vi "subVI Write to Exfo.vi"(2 "error in":errorcluster, 3 "Command Parameter":u16, 4 "Command Number":u8, 5 "VISA Resource Name":refnum<visa-resource-name>) -> (0 "error out":errorcluster, 1 "dup VISA resource name":refnum<visa-resource-name>)   [LabVIEW 2012]
panel:
  # "Output from subVI"
  # "Inputs to SubVI"
  # "1  =  Connect\n2  =  Lock Front Panel\n3  =  Unlock Front Panel\n4  =  Get Software Version\n5  =  Get Lamp Hours\n6  =  Get Unit Status\n7  =  Clear Alarm\n8  =  Run Timed Exposure\n9  =  Open Shutter\n10 = Close Shutter\n11 = Get Intensity Level\n12  = Set Intensity level\n13 = Get Exposure Level\n14 = Set Exposure Time\n15 = Turn Lamp ON\n16 = Turn Lamp OFF"
  # "0, 1, 2, 3 or 4\n \nseconds * 10"
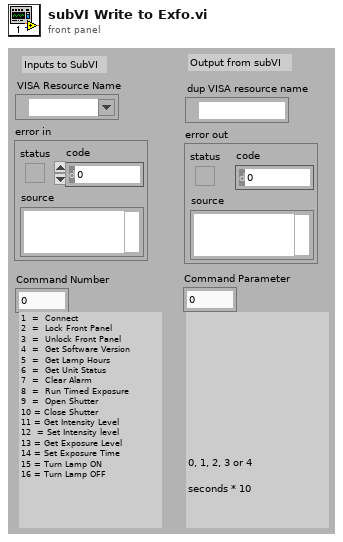
[diagram p1: front panel]
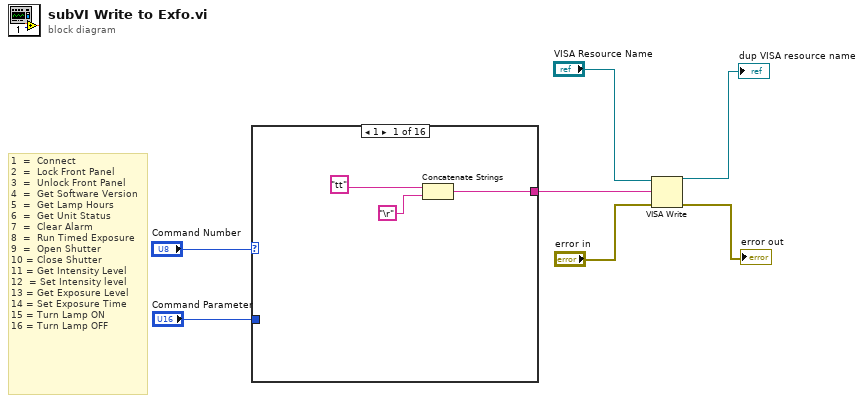
[diagram p0: block diagram]
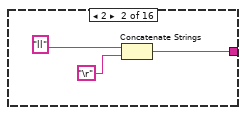
[diagram p2: hidden frame]
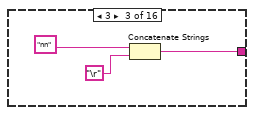
[diagram p3: hidden frame]
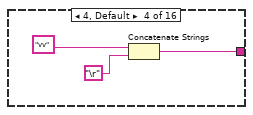
[diagram p4: hidden frame]
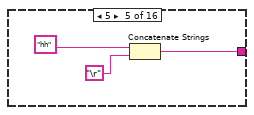
[diagram p5: hidden frame]
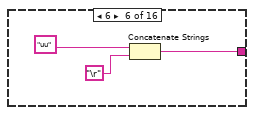
[diagram p6: hidden frame]
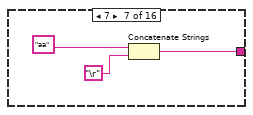
[diagram p7: hidden frame]
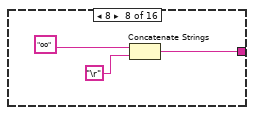
[diagram p8: hidden frame]
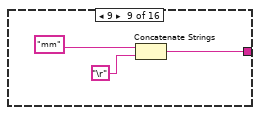
[diagram p9: hidden frame]
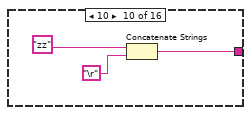
[diagram p10: hidden frame]
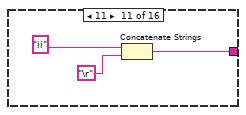
[diagram p11: hidden frame]
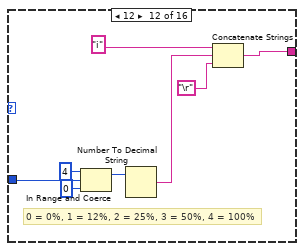
[diagram p12: hidden frame]
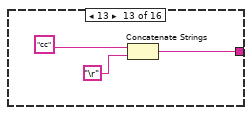
[diagram p13: hidden frame]
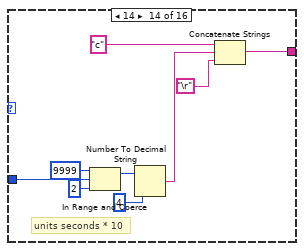
[diagram p14: hidden frame]
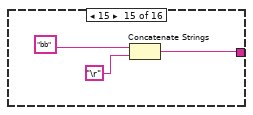
[diagram p15: hidden frame]
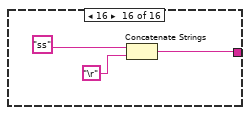
[diagram p16: hidden frame]
diagram:
  # "1  =  Connect\n2  =  Lock Front Panel\n3  =  Unlock Front Panel\n4  =  Get Software Version\n5  =  Get Lamp Hours\n6  =  Get Unit Status\n7  =  Clear Alarm\n8  =  Run Timed Exposure\n9  =  Open Shutter\n10 = Close Shutter\n11 = Get Intensity Level\n12  = Set Intensity level\n13 = Get Exposure Level\n14 = Set Exposure Time\n15 = Turn Lamp ON\n16 = Turn Lamp OFF"
  n1 = case shown="1" "Command Number" {
    tunnel: [w8 w11 w14 w17 w20 w23 w26 w29 w32 w35 w38 w47 w49 w59 w61 w64] -> w4
    tunnel: "Command Parameter" -> [_ _ _ _ _ _ _ _ _ _ _ w46 _ w55 _ _]
    frame 1 {
      n2 = Concatenate Strings("tt" ("string"), "\r") -> (w8:string)
    }
    frame 2 {
      n3 = Concatenate Strings("ll" ("string"), "\r") -> (w11:string)
    }
    frame 3 {
      n4 = Concatenate Strings("nn" ("string"), "\r") -> (w14:string)
    }
    frame 4, Default {
      n5 = Concatenate Strings("vv" ("string"), "\r") -> (w17:string)
    }
    frame 5 {
      n6 = Concatenate Strings("hh" ("string"), "\r") -> (w20:string)
    }
    frame 6 {
      n7 = Concatenate Strings("uu" ("string"), "\r") -> (w23:string)
    }
    frame 7 {
      n8 = Concatenate Strings("aa" ("string"), "\r") -> (w26:string)
    }
    frame 8 {
      n9 = Concatenate Strings("oo" ("string"), "\r") -> (w29:string)
    }
    frame 9 {
      n10 = Concatenate Strings("mm" ("string"), "\r") -> (w32:string)
    }
    frame 10 {
      n11 = Concatenate Strings("zz" ("string"), "\r") -> (w35:string)
    }
    frame 11 {
      n12 = Concatenate Strings("ii" ("string"), "\r") -> (w38:string)
    }
    frame 12 {
      # "0 = 0%, 1 = 12%, 2 = 25%, 3 = 50%, 4 = 100%"
      n13 = In Range and Coerce(upper limit=u8 4, x=w46, lower limit=u8 0) -> (coerced(x)=w43:u16)  [unwired: 1 out]
      n14 = Number To Decimal String(number=w43) -> (decimal integer string=w42:string)  [unwired: 1 out]
      n15 = Concatenate Strings("i" ("string"), w42, "\r") -> (w47:string)
    }
    frame 13 {
      n16 = Concatenate Strings("cc" ("string"), "\r") -> (w49:string)
    }
    frame 14 {
      # "units seconds * 10"
      n17 = In Range and Coerce(upper limit=u16 9999, x=w55, lower limit=u16 2) -> (coerced(x)=w58:u16)  [unwired: 1 out]
      n18 = Number To Decimal String(number=w58, width (-)=i16 4) -> (decimal integer string=w57:string)
      n19 = Concatenate Strings("c" ("string"), w57, "\r") -> (w59:string)
    }
    frame 15 {
      n20 = Concatenate Strings("bb" ("string"), "\r") -> (w61:string)
    }
    frame 16 {
      n21 = Concatenate Strings("ss" ("string"), "\r") -> (w64:string)
    }
  }
  n22 = VISA Write(VISA resource name="VISA Resource Name", write buffer=w4, error in (no error)="error in") -> (VISA resource name out=→"dup VISA resource name":refnum<visa-resource-name>, error out=→"error out":errorcluster)  [unwired: 1 out]
